vi "mWADC_ADC_DATA Record.vi"(8 "Record_Stop":bool, 10 "MW_ADC":refnum<visa-resource-name>) -> (0 "error out":errorcluster, 1 "Data Recording":bool)   [LabVIEW 2019]
uses:
  <vilib>/Utility/file.llb/Write Delimited Spreadsheet (I64).vi
panel:
  out "ADC Count":i32
  in  "Record_Start":bool
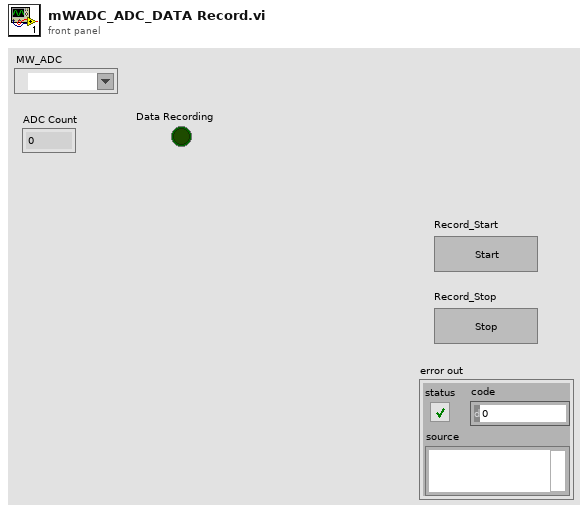
[diagram p1: front panel]
types:
  T1 = enum16{"open", "replace", "create", "open or create", "replace or create", "replace or create with confirmation"}
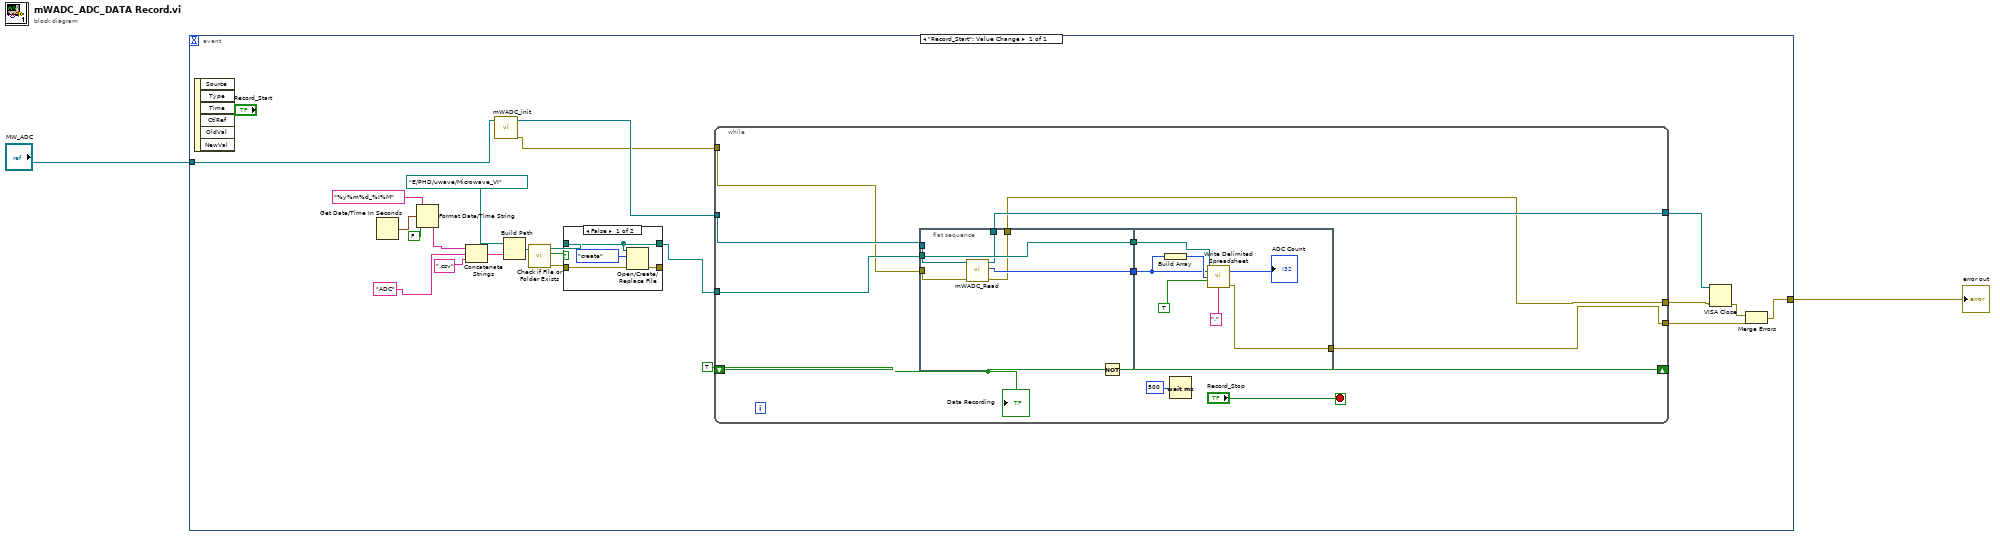
[diagram p0: block diagram]
diagram:
  n1 = event shown="[0] \"Record_Start\": Value Change" {
    selector: _ -> [_]
    dyn-events: _ -> [_]
    timeout: _ -> [_]
    tunnel: "MW_ADC" -> [w11]
    tunnel: [w5] -> w1
    event "Record_Start": Value Change {
      n2 = event-data() -> ()  [unwired: 1 in, 6 out]
      n3 = Get Date/Time In Seconds() -> (seconds since 1Jan1904=w17:timestamp)
      n4 = Format Date/Time String(time format string (%c)="%y%m%d_%I%M", seconds (now)=w17, UTC format=FALSE) -> (date/time string=w14:string)
      n5 = Concatenate Strings(w14, "ADC" ("string"), ".csv" ("string")) -> (w23:string)
      n6 = call "mWADC_init.vi"("mWADC_Port"=w11) -> ("error out"=w9:errorcluster, "reference out"=w10:refnum<visa-resource-name>)  [unwired: 9 in]
      n7 = Build Path(base path=path "E:/PHD/uwave/Microwave_VI" ("path"), name or relative path=w23) -> (appended path=w22:path)
      n8 = call <vilib>:"Check if File or Folder Exists.vi"("path"=w22) -> ("error out"=w20:errorcluster, "file or folder exists?"=w19:bool, "dup path"=w21:path)  [unwired: 8 in]
      n9 = case shown="False" w19 {
        tunnel: w21 -> [w50 w53]
        tunnel: [w51 w54] -> _
        tunnel: [w50 w53] -> w12
        tunnel: w20 -> [w49 w54]
        frame False {
          n10 = Open/Create/Replace File(file path (use dialog)=w50, error in=w49, operation (0:open)=T1."create") -> (error out=w51:errorcluster)  [unwired: 3 in, 2 out]
        }
        frame True {
        }
      }
      n11 = while {
        shift-right: [w36] -> _
        shift-left: TRUE ("x") -> [w35]
        tunnel: w12 -> [w33]
        tunnel: [w28] -> w3
        tunnel: w10 -> [w32]
        tunnel: [w31] -> w8
        tunnel: w9 -> [w30]
        tunnel: [w29] -> w7
        stop <- "Record_Stop" stop-if-true
        n12 = flat-sequence {
          tunnel: [w42] -> w27
          tunnel: w32 -> [w41]
          tunnel: [w40] -> w26
          tunnel: [w39] -> w31
          tunnel: w30 -> [w38]
          tunnel: [w37] -> w29
          tunnel: w33 -> [w42]
          tunnel: w27 -> [w48]
          tunnel: w26 -> [w43]
          tunnel: [w44] -> w28
          frame #0 {
            n13 = call "mWADC_Read.vi"("error in (no error)"=w38, "MW_ADC"=w41) -> ("error out"=w37:errorcluster, "ADC Count"=w40:i32, "VISA resource name out"=w39:refnum<visa-resource-name>)  [unwired: 7 in]
          }
          frame #1 {
            n14 = Build Array(w43) -> (w45:i32[])
            n15 = call-poly <vilib>:"Write Delimited Spreadsheet.vi"("file path (dialog if empty)"=w48, "1D data"=w45, "append to file? (new file:F)"=TRUE, "delimiter (\\t)"="," ("delimiter (\\t)")) -> ("error out"=w44:errorcluster)  [unwired: 10 in, 1 out]
            "ADC Count" <- w43
          }
        }
        n16 = Not(x=w35) -> (.not. x?=w36:bool)
        n17 = Wait (ms)(milliseconds to wait=u32 500) -> ()  [unwired: 1 out]
        "Data Recording" <- w35
      }
      n18 = VISA Close(VISA resource name=w8, error in (no error)=w7) -> (error out=w6:errorcluster)
      n19 = Merge Errors(w6, w3) -> (w5:errorcluster)
    }
  }
  "error out" <- w1
